vi "get_base.vi"(1 "T":T1) -> (0 "Array":dbl[](array[numeric]))   [LabVIEW 2013]
uses:
  <vilib>/Analysis/Matrix/Datatypes/RealMatrix.ctl
  <vilib>/Analysis/Matrix/NI_Matrix.lvlib
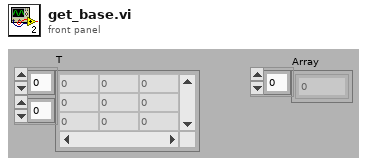
[diagram p1: front panel]
types:
  T1 = typedef "NI_Matrix.lvlib/RealMatrix.ctl" = dbl[][]
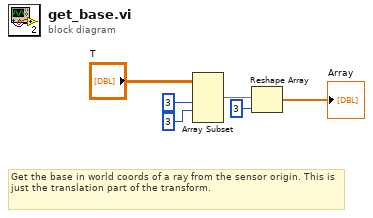
[diagram p0: block diagram]
diagram:
  # "Get the base in world coords of a ray from the sensor origin. This is just the translation part of the transform."
  n1 = Array Subset(array="T", length (row)=3 ("length"), index (col)=3 ("index")) -> (w4:T1)  [unwired: 2 in]
  n2 = Reshape Array(w4, 3 ("dimension size")) -> (→"Array":dbl[])
